vi "CRYGet Title Name and Icon from Type.vi"() -> (2 "Icon Name":string, 3 "Title No":i32)   [LabVIEW 2013]
uses:
  Global/CRYCurve Library Global.vi
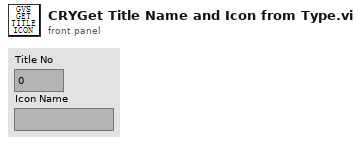
[diagram p1: front panel]
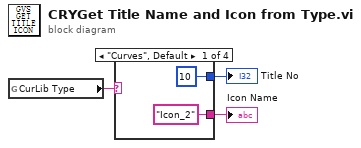
[diagram p0: block diagram]
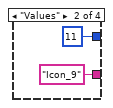
[diagram p2: hidden frame]
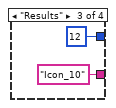
[diagram p3: hidden frame]
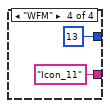
[diagram p4: hidden frame]
diagram:
  n1 = global read "CRYCurve Library Global.vi" "CurLib Type"() -> (w3:string)
  n2 = case shown="\"Curves\", Default" w3 {
    tunnel: [10 ("Error No") 11 ("Error No") 12 ("Error No") 13 ("Error No")] -> w2
    tunnel: ["Icon_2" ("sIcon_Out") "Icon_9" ("sIcon_Out") "Icon_10" ("sIcon_Out") "Icon_11" ("sIcon_Out")] -> w1
    frame "Curves", Default {
    }
    frame "Values" {
    }
    frame "Results" {
    }
    frame "WFM" {
    }
  }
  "Title No" <- w2
  "Icon Name" <- w1
